vi "LowPassFilterOma_2.vi"(10 "Angle_y_2":dbl, 11 "Angle_x_2":dbl) -> (2 "y_filt_2":dbl, 3 "x_filt_2":dbl)   [LabVIEW 2016]
uses:
  <vilib>/ptbypt/NI_PtbyPt.lvlib
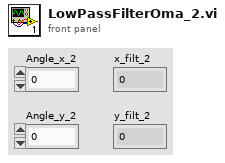
[diagram p1: front panel]
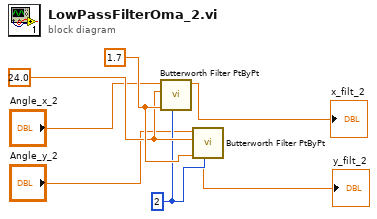
[diagram p0: block diagram]
diagram:
  w7 = 1.7 ("low cutoff freq: fl")
  w6 = 24.0 ("sampling freq: fs")
  w5 = 2 ("order")
  n1 = call <vilib>:"Butterworth Filter PtByPt.vi"("order"=w5, "low cutoff freq: fl"=w7, "sampling freq: fs"=w6, "x"="Angle_x_2") -> ("Filtered x"=→"x_filt_2":dbl)  [unwired: 5 in, 1 out]
  n2 = call <vilib>:"Butterworth Filter PtByPt.vi"("order"=w5, "low cutoff freq: fl"=w7, "sampling freq: fs"=w6, "x"="Angle_y_2") -> ("Filtered x"=→"y_filt_2":dbl)  [unwired: 5 in, 1 out]
